vi "globalTearDown.vi"(8 "error in":errorcluster, 11 "cRIO System Tests in":refnum<class "cRIO System Tests.lvclass">) -> (0 "error out":errorcluster, 3 "cRIO System Tests out":refnum<class "cRIO System Tests.lvclass">)   [LabVIEW 2020, in "cRIO System Tests.lvclass"]
uses:
  cRIO System Tests.lvclass
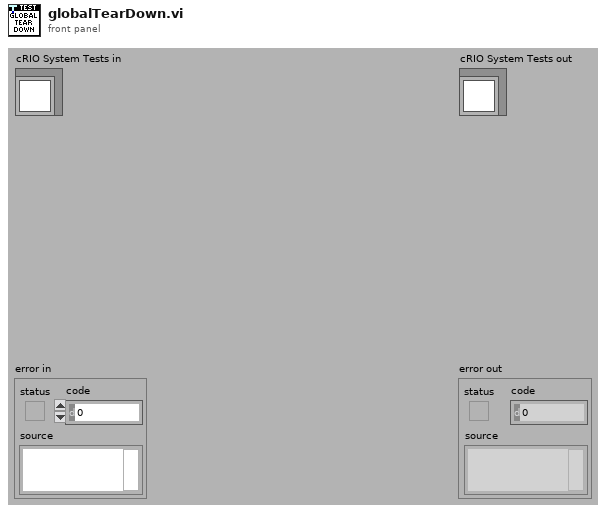
[diagram p1: front panel]
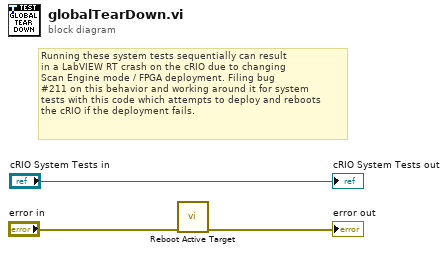
[diagram p0: block diagram]
diagram:
  # "Running these system tests sequentially can result\nin a LabVIEW RT crash on the cRIO due to changing\nScan Engine mode / FPGA deployment. Filing bug\n#211 on this behavior and working around it for system\ntests with this code which attempts to deploy and reboots\nthe cRIO if the deployment fails."
  n1 = call "Reboot Active Target.vi"("error in"="error in") -> ("error out"=→"error out":errorcluster)  [unwired: 10 in]
  "cRIO System Tests out" <- "cRIO System Tests in"
